vi "Channel Play.vi"(8 "error in (no error)":errorcluster, 10 "Channel Index":i32, 11 "Mixer in":refnum<class "Mixer.lvclass">) -> (0 "error out":errorcluster, 3 "Mixer out":refnum<class "Mixer.lvclass">)   [LabVIEW 2020, in "G-Audio.lvlib" / "Mixer.lvclass"]
doc: "Playback the specified channel.\n\nResumes playback if the channel is paused. If the channel is already playing, resets the playback position to zero and continues playing.\n\nOnly applies if channel state is not Empty or Loading."
uses:
  Mixer.lvclass
  Controls/Message.ctl
  Controls/Command.ctl
  Mixer.lvclass/Mixer.ctl
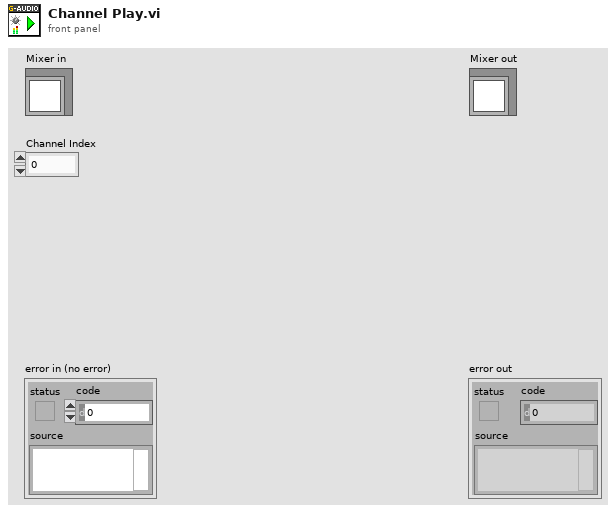
[diagram p1: front panel]
types:
  T1 = typedef "G-Audio.lvlib/Mixer.lvclass/Message.ctl" = cluster{"Command":T2, "Channel":i32, "Payload":variant}
  T2 = typedef "G-Audio.lvlib/Mixer.lvclass/Command.ctl" = enum16{"Channel Stop", "Channel Pause", "Channel Play", "Channel Volume"}
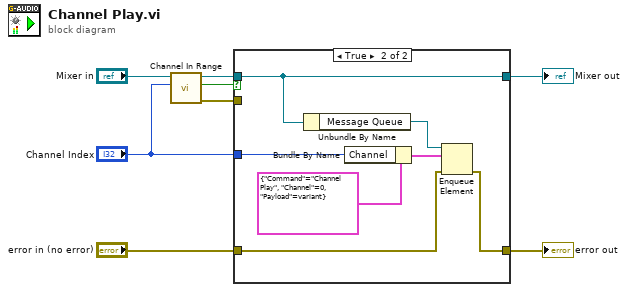
[diagram p0: block diagram]
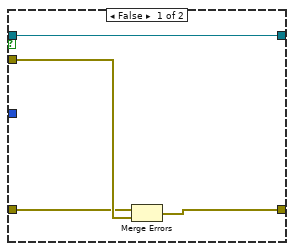
[diagram p2: hidden frame]
diagram:
  n1 = call "Channel In Range.vi"("Channel Index"="Channel Index", "Mixer in"="Mixer in") -> ("error out"=w1:errorcluster, "In Range"=w2:bool, "Mixer out"=w4:refnum<class "Mixer.lvclass">)  [unwired: 7 in]
  n2 = case shown="True" w2 {
    tunnel: w4 -> [w12 w13]
    tunnel: "Channel Index" -> [_ w16]
    tunnel: "error in (no error)" -> [w10 w15]
    tunnel: [w9 w14] -> w6
    tunnel: [w12 w13] -> w5
    tunnel: w1 -> [w11 _]
    frame False {
      n3 = Merge Errors(w10, w11) -> (w9:errorcluster)
    }
    frame True {
      n4 = Unbundle By Name(w13) -> ("Message Queue"=w19:refnum<queue>)
      n5 = Bundle By Name(cluster=T1 {"Command"=enum."Channel Play", "Channel"=0, "Payload"=variant} ("element"), "Channel"=w16) -> (w17:T1)
      n6 = Enqueue Element(queue=w19, element=w17, error in (no error)=w15) -> (error out=w14:errorcluster)  [unwired: 1 in, 2 out]
    }
  }
  "error out" <- w6
  "Mixer out" <- w5
